vi "Step Flow.vi"(8 "error in (no error)":errorcluster, 11 "Conditional Jump Step in":refnum<class "Conditional Jump Step.lvclass">) -> (0 "error out":errorcluster, 3 "Conditional Jump Step out":refnum<class "Conditional Jump Step.lvclass">)   [LabVIEW 2015, in "Conditional Jump Step.lvclass"]
uses:
  Conditional Jump Step.lvclass
  classes/Step/Execution/Step State Enum.ctl
  classes/Step/Execution/Step.lvclass
  classes/Step/Execution/Step Flow Control.ctl
  classes/Step/Execution/StepState.ctl
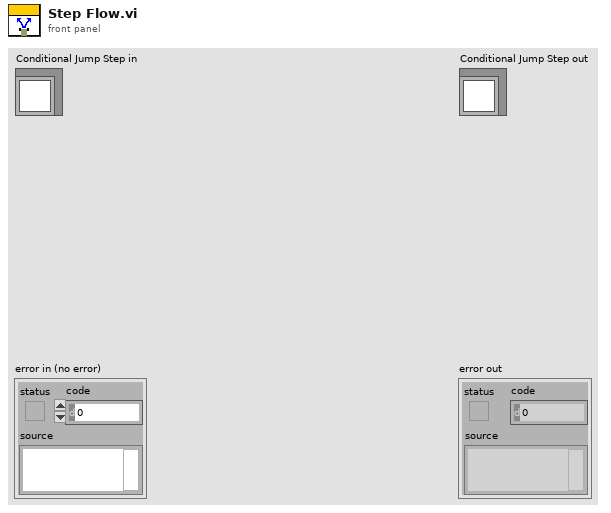
[diagram p1: front panel]
types:
  T1 = typedef "Step.lvclass/Step Flow Control.ctl" = enum16{"Next Step", "Jump"}
  T2 = typedef "Step.lvclass/StepState.ctl" = cluster{"Step State":T3, "Flow Control":T1, "Jump Index":i32}
  T3 = typedef "Step.lvclass/Step State Enum.ctl" = enum16{"Start", "Skipped", "Timeout", "Completed", "Running", "Aborted"}
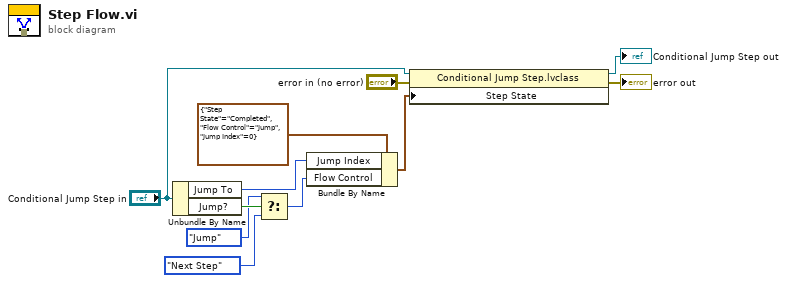
[diagram p0: block diagram]
diagram:
  n1 = Unbundle By Name("Conditional Jump Step in") -> ("Jump To"=w6:i32, "Jump?"=w4:bool)
  n2 = Select(t=Step_Flow_Control."Jump" ("Flow Control"), s=w4, f=Step_Flow_Control."Next Step") -> (s? t:f=w1:T1)
  n3 = Bundle By Name(cluster=T2 {"Step State"=enum."Completed", "Flow Control"=enum."Jump", "Jump Index"=0} ("f"), "Jump Index"=w6, "Flow Control"=w1) -> (w5:T2)
  n4 = property class="Conditional Jump Step.lvclass"(reference="Conditional Jump Step in", error in="error in (no error)", "Step State"=w5) -> (reference out=→"Conditional Jump Step out":refnum<class "Conditional Jump Step.lvclass">, error out=→"error out":errorcluster)
